vi "Read Tag Name.vi"(8 "error in (no error)":errorcluster, 11 "XML in":refnum<class "XML.lvclass">) -> (0 "error out":errorcluster, 2 "Tag Name":string, 3 "XML out":refnum<class "XML.lvclass">)   [LabVIEW 2020, in "XML.lvlib" / "XML.lvclass"]
uses:
  <vilib>/gpm_packages/@cs/persistence/source/XML/XML.lvclass
  <vilib>/gpm_packages/@cs/persistence/source/XML/XML.lvclass/XML.ctl
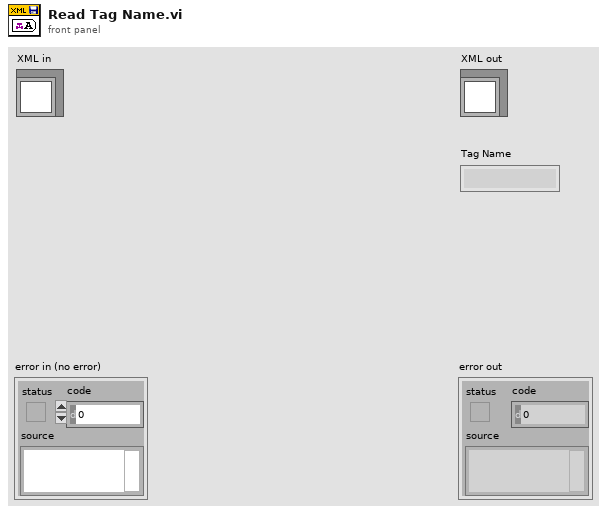
[diagram p1: front panel]
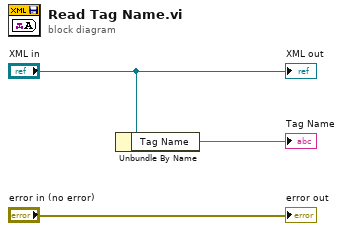
[diagram p0: block diagram]
diagram:
  n1 = Unbundle By Name("XML in") -> ("Tag Name"=→"Tag Name":string)
  "error out" <- "error in (no error)"
  "XML out" <- "XML in"
